vi "UMLEditor Main.vi"(1 "StartProject":string, 3 "StartTarget":string) -> ()   [LabVIEW 2012] (continued)
            n1211 = event-data() -> ()  [unwired: 2 out]
            n1212 = Unbundle By Name(w3369) -> ("ToolHelp"=w3371:bool)
            n1213 = local read "Help"() -> (w3370:bool)
            n1214 = And(x=w3371, y=w3370) -> (x .and. y?=w3368:bool)
            n1215 = case shown="True" w3368 {
              tunnel: w3373 -> [w3374 w3376]
              tunnel: [w3374 w3375] -> w3372
              tunnel: w3369 -> [_ _]
              frame False {
              }
              frame True {
                n1216 = call <resource>:"ContextHelp_HelpTexts.vi"("HelpText (enum or string)"=ContextHelp_HelpTexts."BClass" ("HelpText")) -> ("HelpOut"=w3378:T57)  [unwired: 18 out]
                n1217 = call <resource>:"ContextHelp_SendMessageToPopUp.vi"("PopUpMessage"=w3378, "error in (no error)"=w3376) -> ("error out"=w3375:errorcluster)  [unwired: 1 in, 16 out]
              }
            }
          }
          event Mouse Enter {
            n1218 = event-data() -> ()  [unwired: 2 out]
            n1219 = Unbundle By Name(w3379) -> ("ToolHelp"=w3382:bool)
            n1220 = local read "Help"() -> (w3381:bool)
            n1221 = And(x=w3382, y=w3381) -> (x .and. y?=w3380:bool)
            n1222 = case shown="True" w3380 {
              tunnel: w3384 -> [w3385 w3387]
              tunnel: [w3385 w3386] -> w3383
              tunnel: w3379 -> [_ _]
              frame False {
              }
              frame True {
                n1223 = call <resource>:"ContextHelp_HelpTexts.vi"("HelpText (enum or string)"=ContextHelp_HelpTexts."BInterface" ("HelpText")) -> ("HelpOut"=w3389:T57)  [unwired: 18 out]
                n1224 = call <resource>:"ContextHelp_SendMessageToPopUp.vi"("PopUpMessage"=w3389, "error in (no error)"=w3387) -> ("error out"=w3386:errorcluster)  [unwired: 1 in, 16 out]
              }
            }
          }
          event Mouse Enter {
            n1225 = event-data() -> ()  [unwired: 2 out]
            n1226 = Unbundle By Name(w3391) -> ("ToolHelp"=w3393:bool)
            n1227 = local read "Help"() -> (w3392:bool)
            n1228 = And(x=w3393, y=w3392) -> (x .and. y?=w3390:bool)
            n1229 = case shown="True" w3390 {
              tunnel: w3395 -> [w3396 w3398]
              tunnel: [w3396 w3397] -> w3394
              tunnel: w3391 -> [_ _]
              frame False {
              }
              frame True {
                n1230 = call <resource>:"ContextHelp_HelpTexts.vi"("HelpText (enum or string)"=ContextHelp_HelpTexts."BPackage" ("HelpText")) -> ("HelpOut"=w3400:T57)  [unwired: 18 out]
                n1231 = call <resource>:"ContextHelp_SendMessageToPopUp.vi"("PopUpMessage"=w3400, "error in (no error)"=w3398) -> ("error out"=w3397:errorcluster)  [unwired: 1 in, 16 out]
              }
            }
          }
          event Mouse Enter {
            n1232 = event-data() -> ()  [unwired: 2 out]
            n1233 = Unbundle By Name(w3401) -> ("ToolHelp"=w3404:bool)
            n1234 = local read "Help"() -> (w3403:bool)
            n1235 = And(x=w3404, y=w3403) -> (x .and. y?=w3402:bool)
            n1236 = case shown="True" w3402 {
              tunnel: w3406 -> [w3407 w3409]
              tunnel: [w3407 w3408] -> w3405
              tunnel: w3401 -> [_ _]
              frame False {
              }
              frame True {
                n1237 = call <resource>:"ContextHelp_HelpTexts.vi"("HelpText (enum or string)"=ContextHelp_HelpTexts."BDependency" ("HelpText")) -> ("HelpOut"=w3411:T57)  [unwired: 18 out]
                n1238 = call <resource>:"ContextHelp_SendMessageToPopUp.vi"("PopUpMessage"=w3411, "error in (no error)"=w3409) -> ("error out"=w3408:errorcluster)  [unwired: 1 in, 16 out]
              }
            }
          }
          event Mouse Enter {
            n1239 = event-data() -> ()  [unwired: 2 out]
            n1240 = Unbundle By Name(w3412) -> ("ToolHelp"=w3415:bool)
            n1241 = local read "Help"() -> (w3414:bool)
            n1242 = And(x=w3415, y=w3414) -> (x .and. y?=w3413:bool)
            n1243 = case shown="True" w3413 {
              tunnel: w3417 -> [w3418 w3420]
              tunnel: [w3418 w3419] -> w3416
              tunnel: w3412 -> [_ _]
              frame False {
              }
              frame True {
                n1244 = call <resource>:"ContextHelp_HelpTexts.vi"("HelpText (enum or string)"=ContextHelp_HelpTexts."BInheritance" ("HelpText")) -> ("HelpOut"=w3422:T57)  [unwired: 18 out]
                n1245 = call <resource>:"ContextHelp_SendMessageToPopUp.vi"("PopUpMessage"=w3422, "error in (no error)"=w3420) -> ("error out"=w3419:errorcluster)  [unwired: 1 in, 16 out]
              }
            }
          }
          event Mouse Enter {
            n1246 = event-data() -> ()  [unwired: 2 out]
            n1247 = Unbundle By Name(w3423) -> ("ToolHelp"=w3426:bool)
            n1248 = local read "Help"() -> (w3425:bool)
            n1249 = And(x=w3426, y=w3425) -> (x .and. y?=w3424:bool)
            n1250 = case shown="True" w3424 {
              tunnel: w3428 -> [w3429 w3431]
              tunnel: [w3429 w3430] -> w3427
              tunnel: w3423 -> [_ _]
              frame False {
              }
              frame True {
                n1251 = call <resource>:"ContextHelp_HelpTexts.vi"("HelpText (enum or string)"=ContextHelp_HelpTexts."BInterfaceImplementation" ("HelpText")) -> ("HelpOut"=w3433:T57)  [unwired: 18 out]
                n1252 = call <resource>:"ContextHelp_SendMessageToPopUp.vi"("PopUpMessage"=w3433, "error in (no error)"=w3431) -> ("error out"=w3430:errorcluster)  [unwired: 1 in, 16 out]
              }
            }
          }
          event Mouse Enter {
            n1253 = event-data() -> ()  [unwired: 2 out]
            n1254 = Unbundle By Name(w3434) -> ("ToolHelp"=w3437:bool)
            n1255 = local read "Help"() -> (w3436:bool)
            n1256 = And(x=w3437, y=w3436) -> (x .and. y?=w3435:bool)
            n1257 = case shown="True" w3435 {
              tunnel: w3439 -> [w3440 w3442]
              tunnel: [w3440 w3441] -> w3438
              tunnel: w3434 -> [_ _]
              frame False {
              }
              frame True {
                n1258 = call <resource>:"ContextHelp_HelpTexts.vi"("HelpText (enum or string)"=ContextHelp_HelpTexts."BAssociation" ("HelpText")) -> ("HelpOut"=w3444:T57)  [unwired: 18 out]
                n1259 = call <resource>:"ContextHelp_SendMessageToPopUp.vi"("PopUpMessage"=w3444, "error in (no error)"=w3442) -> ("error out"=w3441:errorcluster)  [unwired: 1 in, 16 out]
              }
            }
          }
          event Mouse Enter {
            n1260 = event-data() -> ()  [unwired: 2 out]
            n1261 = Unbundle By Name(w3446) -> ("ToolHelp"=w3448:bool)
            n1262 = local read "Help"() -> (w3447:bool)
            n1263 = And(x=w3448, y=w3447) -> (x .and. y?=w3445:bool)
            n1264 = case shown="True" w3445 {
              tunnel: w3450 -> [w3451 w3453]
              tunnel: [w3451 w3452] -> w3449
              tunnel: w3446 -> [_ _]
              frame False {
              }
              frame True {
                n1265 = call <resource>:"ContextHelp_HelpTexts.vi"("HelpText (enum or string)"=ContextHelp_HelpTexts."BAggregation" ("HelpText")) -> ("HelpOut"=w3455:T57)  [unwired: 18 out]
                n1266 = call <resource>:"ContextHelp_SendMessageToPopUp.vi"("PopUpMessage"=w3455, "error in (no error)"=w3453) -> ("error out"=w3452:errorcluster)  [unwired: 1 in, 16 out]
              }
            }
          }
          event Mouse Enter {
            n1267 = event-data() -> ()  [unwired: 2 out]
            n1268 = Unbundle By Name(w3456) -> ("ToolHelp"=w3459:bool)
            n1269 = local read "Help"() -> (w3458:bool)
            n1270 = And(x=w3459, y=w3458) -> (x .and. y?=w3457:bool)
            n1271 = case shown="False" w3457 {
              tunnel: w3461 -> [w3462 w3464]
              tunnel: [w3462 w3463] -> w3460
              tunnel: w3456 -> [_ _]
              frame False {
              }
              frame True {
                n1272 = call <resource>:"ContextHelp_HelpTexts.vi"("HelpText (enum or string)"=ContextHelp_HelpTexts."BCompAggregation" ("HelpText")) -> ("HelpOut"=w3466:T57)  [unwired: 18 out]
                n1273 = call <resource>:"ContextHelp_SendMessageToPopUp.vi"("PopUpMessage"=w3466, "error in (no error)"=w3464) -> ("error out"=w3463:errorcluster)  [unwired: 1 in, 16 out]
              }
            }
          }
          event Mouse Enter {
            # "Object"
            n1274 = event-data() -> ()  [unwired: 3 out]
            n1275 = Unbundle By Name(w3468) -> ("ToolHelp"=w3470:bool)
            n1276 = local read "Help"() -> (w3469:bool)
            n1277 = And(x=w3470, y=w3469) -> (x .and. y?=w3467:bool)
            n1278 = case shown="True" w3467 {
              tunnel: w3472 -> [w3473 w3475]
              tunnel: [w3473 w3474] -> w3471
              tunnel: w3468 -> [_ _]
              frame False {
              }
              frame True {
                n1279 = call <resource>:"ContextHelp_HelpTexts.vi"("HelpText (enum or string)"=ContextHelp_HelpTexts."BSystem" ("HelpText")) -> ("HelpOut"=w3477:T57)  [unwired: 18 out]
                n1280 = call <resource>:"ContextHelp_SendMessageToPopUp.vi"("PopUpMessage"=w3477, "error in (no error)"=w3475) -> ("error out"=w3474:errorcluster)  [unwired: 1 in, 16 out]
              }
            }
          }
          event Mouse Enter {
            # "Object"
            n1281 = event-data() -> ()  [unwired: 3 out]
            n1282 = Unbundle By Name(w3479) -> ("ToolHelp"=w3481:bool)
            n1283 = local read "Help"() -> (w3480:bool)
            n1284 = And(x=w3481, y=w3480) -> (x .and. y?=w3478:bool)
            n1285 = case shown="True" w3478 {
              tunnel: w3483 -> [w3484 w3486]
              tunnel: [w3484 w3485] -> w3482
              tunnel: w3479 -> [_ _]
              frame False {
              }
              frame True {
                n1286 = call <resource>:"ContextHelp_HelpTexts.vi"("HelpText (enum or string)"=ContextHelp_HelpTexts."BActor" ("HelpText")) -> ("HelpOut"=w3488:T57)  [unwired: 18 out]
                n1287 = call <resource>:"ContextHelp_SendMessageToPopUp.vi"("PopUpMessage"=w3488, "error in (no error)"=w3486) -> ("error out"=w3485:errorcluster)  [unwired: 1 in, 16 out]
              }
            }
          }
          event Mouse Enter {
            # "Object"
            n1288 = event-data() -> ()  [unwired: 3 out]
            n1289 = Unbundle By Name(w3490) -> ("ToolHelp"=w3492:bool)
            n1290 = local read "Help"() -> (w3491:bool)
            n1291 = And(x=w3492, y=w3491) -> (x .and. y?=w3489:bool)
            n1292 = case shown="True" w3489 {
              tunnel: w3494 -> [w3495 w3497]
              tunnel: [w3495 w3496] -> w3493
              tunnel: w3490 -> [_ _]
              frame False {
              }
              frame True {
                n1293 = call <resource>:"ContextHelp_HelpTexts.vi"("HelpText (enum or string)"=ContextHelp_HelpTexts."BUseCase" ("HelpText")) -> ("HelpOut"=w3499:T57)  [unwired: 18 out]
                n1294 = call <resource>:"ContextHelp_SendMessageToPopUp.vi"("PopUpMessage"=w3499, "error in (no error)"=w3497) -> ("error out"=w3496:errorcluster)  [unwired: 1 in, 16 out]
              }
            }
          }
          event Mouse Enter {
            # "Object"
            n1295 = event-data() -> ()  [unwired: 3 out]
            n1296 = Unbundle By Name(w3501) -> ("ToolHelp"=w3503:bool)
            n1297 = local read "Help"() -> (w3502:bool)
            n1298 = And(x=w3503, y=w3502) -> (x .and. y?=w3500:bool)
            n1299 = case shown="True" w3500 {
              tunnel: w3505 -> [w3506 w3508]
              tunnel: [w3506 w3507] -> w3504
              tunnel: w3501 -> [_ _]
              frame False {
              }
              frame True {
                n1300 = call <resource>:"ContextHelp_HelpTexts.vi"("HelpText (enum or string)"=ContextHelp_HelpTexts."BUseCaseDiagramAssociation" ("HelpText")) -> ("HelpOut"=w3510:T57)  [unwired: 18 out]
                n1301 = call <resource>:"ContextHelp_SendMessageToPopUp.vi"("PopUpMessage"=w3510, "error in (no error)"=w3508) -> ("error out"=w3507:errorcluster)  [unwired: 1 in, 16 out]
              }
            }
          }
          event Mouse Enter {
            # "Object"
            n1302 = event-data() -> ()  [unwired: 3 out]
            n1303 = Unbundle By Name(w3512) -> ("ToolHelp"=w3514:bool)
            n1304 = local read "Help"() -> (w3513:bool)
            n1305 = And(x=w3514, y=w3513) -> (x .and. y?=w3511:bool)
            n1306 = case shown="True" w3511 {
              tunnel: w3516 -> [w3517 w3519]
              tunnel: [w3517 w3518] -> w3515
              tunnel: w3512 -> [_ _]
              frame False {
              }
              frame True {
                n1307 = call <resource>:"ContextHelp_HelpTexts.vi"("HelpText (enum or string)"=ContextHelp_HelpTexts."BIncludes" ("HelpText")) -> ("HelpOut"=w3521:T57)  [unwired: 18 out]
                n1308 = call <resource>:"ContextHelp_SendMessageToPopUp.vi"("PopUpMessage"=w3521, "error in (no error)"=w3519) -> ("error out"=w3518:errorcluster)  [unwired: 1 in, 16 out]
              }
            }
          }
          event Mouse Enter {
            # "Object"
            n1309 = event-data() -> ()  [unwired: 3 out]
            n1310 = Unbundle By Name(w3523) -> ("ToolHelp"=w3525:bool)
            n1311 = local read "Help"() -> (w3524:bool)
            n1312 = And(x=w3525, y=w3524) -> (x .and. y?=w3522:bool)
            n1313 = case shown="True" w3522 {
              tunnel: w3527 -> [w3528 w3530]
              tunnel: [w3528 w3529] -> w3526
              tunnel: w3523 -> [_ _]
              frame False {
              }
              frame True {
                n1314 = call <resource>:"ContextHelp_HelpTexts.vi"("HelpText (enum or string)"=ContextHelp_HelpTexts."BExtends" ("HelpText")) -> ("HelpOut"=w3532:T57)  [unwired: 18 out]
                n1315 = call <resource>:"ContextHelp_SendMessageToPopUp.vi"("PopUpMessage"=w3532, "error in (no error)"=w3530) -> ("error out"=w3529:errorcluster)  [unwired: 1 in, 16 out]
              }
            }
          }
          event Mouse Enter {
            # "Object"
            n1316 = event-data() -> ()  [unwired: 3 out]
            n1317 = Unbundle By Name(w3534) -> ("ToolHelp"=w3536:bool)
            n1318 = local read "Help"() -> (w3535:bool)
            n1319 = And(x=w3536, y=w3535) -> (x .and. y?=w3533:bool)
            n1320 = case shown="True" w3533 {
              tunnel: w3538 -> [w3539 w3541]
              tunnel: [w3539 w3540] -> w3537
              tunnel: w3534 -> [_ _]
              frame False {
              }
              frame True {
                n1321 = call <resource>:"ContextHelp_HelpTexts.vi"("HelpText (enum or string)"=ContextHelp_HelpTexts."BGeneralization" ("HelpText")) -> ("HelpOut"=w3543:T57)  [unwired: 18 out]
                n1322 = call <resource>:"ContextHelp_SendMessageToPopUp.vi"("PopUpMessage"=w3543, "error in (no error)"=w3541) -> ("error out"=w3540:errorcluster)  [unwired: 1 in, 16 out]
              }
            }
          }
          event Mouse Enter {
            # "Object"
            n1323 = event-data() -> ()  [unwired: 3 out]
            n1324 = Unbundle By Name(w3545) -> ("ToolHelp"=w3547:bool)
            n1325 = local read "Help"() -> (w3546:bool)
            n1326 = And(x=w3547, y=w3546) -> (x .and. y?=w3544:bool)
            n1327 = case shown="True" w3544 {
              tunnel: w3549 -> [w3550 w3552]
              tunnel: [w3550 w3551] -> w3548
              tunnel: w3545 -> [_ _]
              frame False {
              }
              frame True {
                n1328 = call <resource>:"ContextHelp_HelpTexts.vi"("HelpText (enum or string)"=ContextHelp_HelpTexts."BObject" ("HelpText")) -> ("HelpOut"=w3554:T57)  [unwired: 18 out]
                n1329 = call <resource>:"ContextHelp_SendMessageToPopUp.vi"("PopUpMessage"=w3554, "error in (no error)"=w3552) -> ("error out"=w3551:errorcluster)  [unwired: 1 in, 16 out]
              }
            }
          }
          event Mouse Enter {
            # "Object"
            n1330 = event-data() -> ()  [unwired: 3 out]
            n1331 = Unbundle By Name(w3556) -> ("ToolHelp"=w3558:bool)
            n1332 = local read "Help"() -> (w3557:bool)
            n1333 = And(x=w3558, y=w3557) -> (x .and. y?=w3555:bool)
            n1334 = case shown="True" w3555 {
              tunnel: w3560 -> [w3561 w3563]
              tunnel: [w3561 w3562] -> w3559
              tunnel: w3556 -> [_ _]
              frame False {
              }
              frame True {
                n1335 = call <resource>:"ContextHelp_HelpTexts.vi"("HelpText (enum or string)"=ContextHelp_HelpTexts."BActionBar" ("HelpText")) -> ("HelpOut"=w3565:T57)  [unwired: 18 out]
                n1336 = call <resource>:"ContextHelp_SendMessageToPopUp.vi"("PopUpMessage"=w3565, "error in (no error)"=w3563) -> ("error out"=w3562:errorcluster)  [unwired: 1 in, 16 out]
              }
            }
          }
          event Mouse Enter {
            # "Object"
            n1337 = event-data() -> ()  [unwired: 3 out]
            n1338 = Unbundle By Name(w3567) -> ("ToolHelp"=w3569:bool)
            n1339 = local read "Help"() -> (w3568:bool)
            n1340 = And(x=w3569, y=w3568) -> (x .and. y?=w3566:bool)
            n1341 = case shown="True" w3566 {
              tunnel: w3571 -> [w3572 w3574]
              tunnel: [w3572 w3573] -> w3570
              tunnel: w3567 -> [_ _]
              frame False {
              }
              frame True {
                n1342 = call <resource>:"ContextHelp_HelpTexts.vi"("HelpText (enum or string)"=ContextHelp_HelpTexts."BCall" ("HelpText")) -> ("HelpOut"=w3576:T57)  [unwired: 18 out]
                n1343 = call <resource>:"ContextHelp_SendMessageToPopUp.vi"("PopUpMessage"=w3576, "error in (no error)"=w3574) -> ("error out"=w3573:errorcluster)  [unwired: 1 in, 16 out]
              }
            }
          }
          event Mouse Enter {
            n1344 = event-data() -> ()  [unwired: 2 out]
            n1345 = Unbundle By Name(w3577) -> ("ToolHelp"=w3580:bool)
            n1346 = local read "Help"() -> (w3579:bool)
            n1347 = And(x=w3580, y=w3579) -> (x .and. y?=w3578:bool)
            n1348 = case shown="True" w3578 {
              tunnel: w3582 -> [w3583 w3585]
              tunnel: [w3583 w3584] -> w3581
              tunnel: w3577 -> [_ _]
              frame False {
              }
              frame True {
                n1349 = call <resource>:"ContextHelp_HelpTexts.vi"("HelpText (enum or string)"=ContextHelp_HelpTexts."BNoteConnector" ("HelpText")) -> ("HelpOut"=w3587:T57)  [unwired: 18 out]
                n1350 = call <resource>:"ContextHelp_SendMessageToPopUp.vi"("PopUpMessage"=w3587, "error in (no error)"=w3585) -> ("error out"=w3584:errorcluster)  [unwired: 1 in, 16 out]
              }
            }
          }
          event Mouse Enter {
            n1351 = event-data() -> ()  [unwired: 4 out]
            n1352 = Unbundle By Name(w3588) -> ("ToolHelp"=w3593:bool)
            n1353 = local read "Help"() -> (w3592:bool)
            n1354 = And(x=w3593, y=w3592) -> (x .and. y?=w3591:bool)
            n1355 = case shown="True" w3591 {
              tunnel: w3589 -> [w3594 w3596]
              tunnel: [w3594 w3595] -> w3590
              tunnel: w3588 -> [_ _]
              frame False {
              }
              frame True {
                n1356 = call <resource>:"ContextHelp_HelpTexts.vi"("HelpText (enum or string)"=ContextHelp_HelpTexts."BNote" ("HelpText")) -> ("HelpOut"=w3598:T57)  [unwired: 18 out]
                n1357 = call <resource>:"ContextHelp_SendMessageToPopUp.vi"("PopUpMessage"=w3598, "error in (no error)"=w3596) -> ("error out"=w3595:errorcluster)  [unwired: 1 in, 16 out]
              }
            }
          }
          event Mouse Enter {
            n1358 = event-data() -> ()  [unwired: 4 out]
            n1359 = Unbundle By Name(w3599) -> ("ToolHelp"=w3604:bool)
            n1360 = local read "Help"() -> (w3603:bool)
            n1361 = And(x=w3604, y=w3603) -> (x .and. y?=w3602:bool)
            n1362 = case shown="True" w3602 {
              tunnel: w3600 -> [w3605 w3607]
              tunnel: [w3605 w3606] -> w3601
              tunnel: w3599 -> [_ _]
              frame False {
              }
              frame True {
                n1363 = call <resource>:"ContextHelp_HelpTexts.vi"("HelpText (enum or string)"=ContextHelp_HelpTexts."BState" ("HelpText")) -> ("HelpOut"=w3609:T57)  [unwired: 18 out]
                n1364 = call <resource>:"ContextHelp_SendMessageToPopUp.vi"("PopUpMessage"=w3609, "error in (no error)"=w3607) -> ("error out"=w3606:errorcluster)  [unwired: 1 in, 16 out]
              }
            }
          }
          event Mouse Enter {
            n1365 = event-data() -> ()  [unwired: 4 out]
            n1366 = Unbundle By Name(w3610) -> ("ToolHelp"=w3615:bool)
            n1367 = local read "Help"() -> (w3614:bool)
            n1368 = And(x=w3615, y=w3614) -> (x .and. y?=w3613:bool)
            n1369 = case shown="True" w3613 {
              tunnel: w3611 -> [w3616 w3618]
              tunnel: [w3616 w3617] -> w3612
              tunnel: w3610 -> [_ _]
              frame False {
              }
              frame True {
                n1370 = call <resource>:"ContextHelp_HelpTexts.vi"("HelpText (enum or string)"=ContextHelp_HelpTexts."BInitialState" ("HelpText")) -> ("HelpOut"=w3620:T57)  [unwired: 18 out]
                n1371 = call <resource>:"ContextHelp_SendMessageToPopUp.vi"("PopUpMessage"=w3620, "error in (no error)"=w3618) -> ("error out"=w3617:errorcluster)  [unwired: 1 in, 16 out]
              }
            }
          }
          event Mouse Enter {
            n1372 = event-data() -> ()  [unwired: 4 out]
            n1373 = Unbundle By Name(w3621) -> ("ToolHelp"=w3626:bool)
            n1374 = local read "Help"() -> (w3625:bool)
            n1375 = And(x=w3626, y=w3625) -> (x .and. y?=w3624:bool)
            n1376 = case shown="True" w3624 {
              tunnel: w3622 -> [w3627 w3629]
              tunnel: [w3627 w3628] -> w3623
              tunnel: w3621 -> [_ _]
              frame False {
              }
              frame True {
                n1377 = call <resource>:"ContextHelp_HelpTexts.vi"("HelpText (enum or string)"=ContextHelp_HelpTexts."BFinalState" ("HelpText")) -> ("HelpOut"=w3631:T57)  [unwired: 18 out]
                n1378 = call <resource>:"ContextHelp_SendMessageToPopUp.vi"("PopUpMessage"=w3631, "error in (no error)"=w3629) -> ("error out"=w3628:errorcluster)  [unwired: 1 in, 16 out]
              }
            }
          }
          event Mouse Enter {
            n1379 = event-data() -> ()  [unwired: 4 out]
            n1380 = Unbundle By Name(w3632) -> ("ToolHelp"=w3637:bool)
            n1381 = local read "Help"() -> (w3636:bool)
            n1382 = And(x=w3637, y=w3636) -> (x .and. y?=w3635:bool)
            n1383 = case shown="True" w3635 {
              tunnel: w3633 -> [w3638 w3640]
              tunnel: [w3638 w3639] -> w3634
              tunnel: w3632 -> [_ _]
              frame False {
              }
              frame True {
                n1384 = call <resource>:"ContextHelp_HelpTexts.vi"("HelpText (enum or string)"=ContextHelp_HelpTexts."BStateTransition" ("HelpText")) -> ("HelpOut"=w3642:T57)  [unwired: 18 out]
                n1385 = call <resource>:"ContextHelp_SendMessageToPopUp.vi"("PopUpMessage"=w3642, "error in (no error)"=w3640) -> ("error out"=w3639:errorcluster)  [unwired: 1 in, 16 out]
              }
            }
          }
          event "RevHistory": Mouse Down {
            n1386 = event-data() -> ("Mods.Double Click"=w3643:bool)  [unwired: 1 out]
            n1387 = case shown="True" w3643 {
              tunnel: w3646 -> [w3647 w3650]
              tunnel: [w3647 w3649] -> w3645
              tunnel: w3644 -> [_ w3648]
              frame False {
              }
              frame True {
                n1388 = call <resource>:"UMLEditor RevisionHistory.vi"("localVariables"=w3648, "error in (no error)"=w3650) -> ("error out"=w3649:errorcluster)  [unwired: 17 out]
              }
            }
          }
          event "Project": Value Change {
            n1389 = event-data() -> ()  [unwired: 2 out]
            n1390 = property on="Project" class="Ring (strict)"() -> ("Strings []"=w3662:string[])  [unwired: 2 in, 2 out]
            n1391 = Index Array(array=w3662, index="Project") -> (element=w3655:string)
            n1392 = call <resource>:"UMLEditor_TargetDialog.vi"("error in (no error)"=w3656, "GetProjectRefByName"=w3655) -> ("error out"=w3653:errorcluster, "ProjectFolder"=w3654:path, "TargetIndex"=w3652:u16, "Targets"=w3651:string[])  [unwired: 5 in, 1 out]
            n1393 = call <resource>:"GetRelativePathOption.vi"() -> ("UseProjectFolderAsBasePath"=w3660:bool)  [unwired: 1 in, 18 out]
            n1394 = property on="Target" class="Ring (strict)"("Strings []"=w3651, "Value"=w3652) -> ()  [unwired: 2 in, 2 out]
            n1395 = case shown="True" w3660 {
              tunnel: w3654 -> [_ w3682]
              tunnel: File_StoredPathesActions."Set Path" ("Method (Get Path)") -> [_ w3681]
              frame False {
              }
              frame True {
                n1396 = call <resource>:"File_ApplicationPaths.vi"("PathName"=UMLEditor_StoredPathes."ClassBasePath" ("UMLPathes"), "Path In"=w3682, "Method (Get Path)"=w3681) -> ()  [unwired: 1 in, 16 out]
              }
            }
            n1397 = Unbundle By Name(w3653) -> ("code"=w3658:i32)
            n1398 = case shown="1055" w3658 {
              tunnel: w3653 -> [w3664 _]
              tunnel: [w3664 w3673] -> w3657
              tunnel: w3656 -> [_ w3673]
              frame 0, Default {
              }
              frame 1055 {
                n1399 = call <resource>:"GDSProject_GetProjects.vi"("OpenProjectRef(True)"=FALSE) -> ("Projects"=w3674:string[])  [unwired: 2 in, 16 out]
                n1400 = Index Array(array=w3674) -> (element=w3672:string)  [unwired: 1 in]
                n1401 = stacked-sequence {
                  tunnel: [w3679] -> w3671
                  tunnel: w3672 -> [w3679]
                  frame #0 {
                    n1402 = One Button Dialog(message="The selected project has been closed.\nSelect another one.") -> ()  [unwired: 2 out]
                  }
                }
                n1403 = call <resource>:"UMLEditor_TargetDialog.vi"("GetProjectRefByName"=w3671) -> ("ProjectFolder"=w3665:path, "TargetIndex"=w3670:u16, "Targets"=w3669:string[])  [unwired: 6 in, 2 out]
                n1404 = call <resource>:"GetRelativePathOption.vi"() -> ("UseProjectFolderAsBasePath"=w3667:bool)  [unwired: 1 in, 18 out]
                n1405 = case shown="True" w3667 {
                  tunnel: w3665 -> [_ w3677]
                  tunnel: File_StoredPathesActions."Set Path" ("Method (Get Path)") -> [_ w3676]
                  frame False {
                  }
                  frame True {
                    n1406 = call <resource>:"File_ApplicationPaths.vi"("PathName"=UMLEditor_StoredPathes."ClassBasePath" ("UMLPathes"), "Path In"=w3677, "Method (Get Path)"=w3676) -> ()  [unwired: 1 in, 16 out]
                  }
                }
                n1407 = property on="Project" class="Ring (strict)"("Strings []"=w3674, "Value"=0) -> ()  [unwired: 2 in, 2 out]
                n1408 = property on="Target" class="Ring (strict)"("Strings []"=w3669, "Value"=w3670) -> ()  [unwired: 2 in, 2 out]
              }
            }
          }
          event "Project": Mouse Down? {
            n1409 = event-data() -> ()  [unwired: 2 out]
            n1410 = property on="Project" class="Ring (strict)"() -> ("Strings []"=w3685:string[])  [unwired: 2 in, 2 out]
            n1411 = call <resource>:"UMLEditor getDiagramInfo.vi"("localVariables"=w3694, "error in (no error)"=w3692) -> ("graph"=w3691:refnum<class "Graph.lvclass">, "error out"=w3690:errorcluster)  [unwired: 16 out]
            n1412 = Index Array(array=w3685) -> (element=w3687:string)  [unwired: 1 in]
            n1413 = Empty String/Path?(string/path=w3687) -> (empty?=w3686:bool)
            n1414 = call-dynamic "getNodes.vi"("reference"=w3691, "error in (no error)"=w3690) -> ("nodes"=w3689:refnum<class "AbstractNode.lvclass">[])  [unwired: 15 in, 2 out]
            n1415 = Empty Array?(array=w3689) -> (empty?=w3688:bool)
            n1416 = Or(x=w3688, y=w3686) -> ()  [unwired: 1 out]
            n1417 = case shown="True" TRUE {
              tunnel: w3692 -> [w3697 w3706]
              tunnel: [w3697 w3705] -> w3695
              tunnel: [TRUE ("Discard?") w3704] -> w3693
              tunnel: w3685 -> [_ w3701]
              frame False {
                n1418 = One Button Dialog(message="You are only allowed to change project if the current diagram is empty.") -> ()  [unwired: 2 out]
              }
              frame True {
                n1419 = call <resource>:"GDSProject_GetProjects.vi"("error in (no error)"=w3706, "OpenProjectRef(True)"=FALSE) -> ("Projects"=w3700:string[], "error out"=w3705:errorcluster)  [unwired: 1 in, 15 out]
                n1420 = Index Array(array=w3700) -> (element=w3703:string)  [unwired: 1 in]
                n1421 = Empty String/Path?(string/path=w3703) -> (empty?=w3702:bool)
                n1422 = case shown="True" w3702 {
                  tunnel: [FALSE ("Discard?") TRUE ("Discard?")] -> w3704
                  tunnel: w3700 -> [w3709 _]
                  tunnel: w3701 -> [w3708 _]
                  frame False {
                    n1423 = for {
                      tunnel: w3709 -> [w3711] mode=indexing
                      shift-right: [w3714] -> w3707
                      shift-left: w3708 -> [w3713]
                      n1424 = Search 1D Array(1D array=w3713, element=w3711) -> (index of element=w3712:i32)  [unwired: 1 out]
                      n1425 = case shown="0, Default" w3712 {
                        tunnel: [w3715 w3718] -> w3714
                        tunnel: w3713 -> [w3715 w3717]
                        tunnel: w3711 -> [_ w3716]
                        frame 0, Default {
                        }
                        frame -1 {
                          n1426 = Build Array (concatenate)(w3717, w3716) -> (w3718:string[])
                        }
                      }
                    }
                    n1427 = property on="Project" class="Ring (strict)"("Strings []"=w3707) -> ()  [unwired: 2 in, 2 out]
                  }
                  frame True {
                    n1428 = call "File Dialog"("prompt"="Select a project to open", "button label"="Open", "pattern (all files)"="*.lvproj", "pattern label"="LabVIEW projects") -> ("selected path"=w3719:path, "cancelled"=w3720:bool)  [unwired: 3 in, 7 out]
                    n1429 = case shown="False" w3720 {
                      tunnel: w3719 -> [w3741 _]
                      frame False {
                        n1430 = call <vilib>:"Set Busy.vi"() -> ("error out"=w3735:errorcluster)  [unwired: 4 in, 7 out]
                        n1431 = invoke class="App" method="Project.Open"(error in=w3735, "Path"=w3741) -> ("Project:Open"=w3740:refnum<vi>)  [unwired: 2 in, 3 out]
                        n1432 = invoke class="Project" method="Open Window"(reference=w3740) -> (reference out=w3738:refnum<vi>, error out=w3739:errorcluster)  [unwired: 2 in, 1 out]
                        n1433 = call <resource>:"GetRelativePathOption.vi"() -> ("UseProjectFolderAsBasePath"=w3728:bool)  [unwired: 1 in, 18 out]
                        n1434 = Close Reference(reference=w3738, error in (no error)=w3739) -> (error out=w3737:errorcluster)
                        n1435 = call <resource>:"GDSProject_GetProjects.vi"("error in (no error)"=w3737, "OpenProjectRef(True)"=FALSE) -> ("Projects"=w3736:string[])  [unwired: 1 in, 16 out]
                        n1436 = Index Array(array=w3736) -> (element=w3733:string)  [unwired: 1 in]
                        n1437 = call <resource>:"UMLEditor_TargetDialog.vi"("GetProjectRefByName"=w3733) -> ("error out"=w3732:errorcluster, "ProjectFolder"=w3726:path, "TargetIndex"=w3730:u16, "Targets"=w3731:string[])  [unwired: 6 in, 1 out]
                        n1438 = case shown="True" w3728 {
                          tunnel: w3726 -> [_ w3743]
                          tunnel: File_StoredPathesActions."Set Path" ("Method (Get Path)") -> [_ w3742]
                          frame False {
                          }
                          frame True {
                            n1439 = call <resource>:"File_ApplicationPaths.vi"("PathName"=UMLEditor_StoredPathes."ClassBasePath" ("UMLPathes"), "Path In"=w3743, "Method (Get Path)"=w3742) -> ()  [unwired: 1 in, 16 out]
                          }
                        }
                        n1440 = property on="Target" class="Ring (strict)"("Strings []"=w3731, "Value"=w3730) -> ()  [unwired: 2 in, 2 out]
                        n1441 = Build Array(w3733) -> (w3734:string[])
                        n1442 = property on="Project" class="Ring (strict)"("Strings []"=w3734) -> ()  [unwired: 2 in, 2 out]
                        n1443 = call <vilib>:"Unset Busy.vi"("error in (no error)"=w3732) -> ()  [unwired: 1 in, 10 out]
                      }
                      frame True {
                      }
                    }
                  }
                }
              }
            }
            n1444 = event-data("Discard?"=w3693) -> ()  [unwired: 1 in, 1 out]
          }
          event "ClassAggregationDialog": Value Change {
            n1445 = event-data() -> ()  [unwired: 7 out]
            n1446 = Unbundle By Name("ClassAggregationDialog") -> ("AddAttribute"=w3745:bool)  [unwired: 1 out]
            n1447 = property on="ClassAggregationDialog" class="Clust (strict)"("Visible"=FALSE) -> ()  [unwired: 2 in, 2 out]
            n1448 = call <resource>:"UMLEditor_AggregationClusterDialogControl.vi"("error in (no error)"=w3750, "Action(SelectSelect)"=T22."GetStatus") -> ("StartEndNodes"=w3747:T59, "AddAggregate?"=w3748:bool, "error out"=w3749:errorcluster)  [unwired: 7 in, 8 out]
            n1449 = case shown="True" w3745 {
              tunnel: w3754 -> [w3759 w3769]
              tunnel: w3749 -> [w3760 w3770]
              tunnel: [w3760 w3763] -> w3755
              tunnel: [w3759 w3768] -> w3753
              tunnel: w3752 -> [_ w3765]
              tunnel: w3748 -> [_ w3762]
              tunnel: w3747 -> [_ w3761]
              frame False {
              }
              frame True {
                n1450 = case shown="False" w3762 {
                  tunnel: w3770 -> [w3775 w3781]
                  tunnel: w3769 -> [w3774 w3782]
                  tunnel: [w3773 w3778] -> w3767
                  tunnel: [w3772 w3779] -> w3766
                  tunnel: [w3771 w3780] -> w3764
                  tunnel: w3761 -> [_ w3777]
                  frame True {
                    n1451 = Unbundle By Name(w3774) -> ("selectedEdge"=w3776:refnum<class "AbstractEdge.lvclass">)
                    n1452 = call <resource>:"UMLEditor CreateAggregationAttributes.vi"("ClassAggregation"=w3776, "error in (no error)"=w3775) -> ("NodeModified"=w3771:refnum<class "AbstractNode.lvclass">, "Modified?"=w3773:bool, "error out"=w3772:errorcluster)  [unwired: 15 out]
                  }
                  frame False {
                    n1453 = Unbundle By Name(w3782) -> ()  [unwired: 1 out]
                    n1454 = call <resource>:"UMLEditor RemoveAggregationAttributes.vi"("StartEndNodes"=w3777, "error in (no error)"=w3781) -> ("NodeModified"=w3780:refnum<class "AbstractNode.lvclass">, "Modified?"=w3778:bool, "error out"=w3779:errorcluster)  [unwired: 15 out]
                  }
                }
                n1455 = case shown="True" w3767 {
                  tunnel: w3769 -> [w3784 w3794]
                  tunnel: [w3784 w3793] -> w3768
                  tunnel: w3766 -> [w3783 w3791]
                  tunnel: w3765 -> [_ w3790]
                  tunnel: w3764 -> [_ w3789]
                  tunnel: [w3783 w3786] -> w3763
                  frame False {
                  }
                  frame True {
                    n1456 = Build Array(w3789) -> (w3788:refnum<class "AbstractNode.lvclass">[])
                    n1457 = call-dynamic "layout.vi"("reference"=w3790, "LayoutNodes(Empty=All)"=w3788, "error in (no error)"=w3791) -> ("error out"=w3787:errorcluster)  [unwired: 15 in, 1 out]
                    n1458 = Bundle By Name(cluster=w3794, "modified"=TRUE, "state"=UMLEditor_statesType."Repaint") -> (w3785:T7)
                    n1459 = call <resource>:"UMLEditor setDiagramInfo.vi"("error in (no error)"=w3787, "localVariablesIn"=w3785, "action"=enum16{"Name/Dir", "Unsaved", "Saved"}."Unsaved") -> ("localVariablesOut"=w3793:T7, "error out"=w3786:errorcluster)  [unwired: 2 in, 13 out]
                  }
                }
              }
            }
            n1460 = stacked-sequence {
              tunnel: [T5 {"AddAttribute"=FALSE, "Don'tAddAttribute"=FALSE, "Close"=FALSE, "Text"=""} ("ClassAggregationDialog")] -> w3746
              tunnel: w3745 -> [_]
              frame #0 {
              }
            }
            n1461 = local write "ClassAggregationDialog"(w3746) -> ()
          }
          event "Target": Value Change {
            n1462 = event-data() -> ()  [unwired: 7 out]
            n1463 = property on="Target" class="Ring (strict)"() -> ("Strings []"=w3805:string[], "Value"=w3804:u16)  [unwired: 2 in, 2 out]
            n1464 = property on="Project" class="Ring (strict)"() -> ("Strings []"=w3800:string[], "Value"=w3799:u16)  [unwired: 2 in, 2 out]
            n1465 = Index Array(array=w3805, index=w3804) -> (element=w3803:string)
            n1466 = Index Array(array=w3800, index=w3799) -> (element=w3798:string)
            n1467 = call <resource>:"UMLEditor_TargetDialog.vi"("error in (no error)"=w3802, "Target"=w3803, "GetProjectRefByName"=w3798) -> ("error out"=w3801:errorcluster)  [unwired: 4 in, 4 out]
          }
        }
        n1468 = Unbundle By Name(w278) -> ("Sync"=w270:bool, "state"=w268:T8)
        n1469 = Select(t=UMLEditor_statesType."AutoSync" ("state"), s=w270, f=w268) -> (s? t:f=w269:T8)
      }
      frame "AutoSync" {
        (unwired) UMLEditor_statesType."Idle" ("state")
        # "Have we been idle for a while?\nIf so, do a sync"
        n1470 = Unbundle By Name(w3809) -> ("LastSync"=w3816:timestamp, "SyncTime"=w3815:u32, "ForceSyncNow"=w3817:bool)
        n1471 = Get Date/Time In Seconds() -> (seconds since 1Jan1904=w3807:timestamp)
        n1472 = Subtract(x=w3807, y=w3816) -> (x-y=w3814:dbl)
        n1473 = Subtract(x=w3815, y=w3814) -> (x-y=w3813:dbl)
        n1474 = To Long Integer(number=w3813) -> (32bit integer=w3810:i32)
        n1475 = Max & Min(x=0, y=w3810) -> (max(x,y)=w3806:i32)  [unwired: 1 out]
        n1476 = Equal To 0?(x=w3806) -> (x = 0?=w3811:bool)
        n1477 = Or(x=w3811, y=w3817) -> (x .or. y?=w3818:bool)
        n1478 = case shown="False" w3818 {
          tunnel: w3824 -> [_ _]
          tunnel: w3809 -> [_ w3855]
          tunnel: [_ w3839] -> w3823
          tunnel: w3817 -> [_ w3840]
          tunnel: w3806 -> [w3827 _]
          tunnel: w3809 -> [w3826 w3838]
          tunnel: [w3826 w3837] -> w3808
          tunnel: w3807 -> [_ w3836]
          frame False {
            n1479 = feedback-in #2(w3827) -> ()
            n1480 = feedback #2() -> (w3829:i32)  [unwired: 1 in]
            n1481 = Not Equal?(x=w3829, y=w3827) -> (x != y?=w3828:bool)
            n1482 = case shown="True" w3828 {
              tunnel: w3827 -> [_ w3830]
              frame False {
              }
              frame True {
                n1483 = case shown="1" w3830 {
                  selector: w3830 -> [_ w3833]
                  tunnel: ["Auto sync in 1 second" ("format string") w3834] -> w3831
                  frame 1 {
                  }
                  frame Default {
                    n1484 = Format Into String(format string="Auto sync in %d seconds", w3833) -> (resulting string=w3834:string)  [unwired: 2 in, 1 out]
                  }
                }
                n1485 = local write "StatusBar"(w3831) -> ()
              }
            }
          }
          frame True {
            w3845 = timestamp(0 s since 1904-01-01)
            n1486 = call <resource>:"UMLEditor getDiagramInfo.vi"("localVariables"=w3855) -> ("graph"=w3841:refnum<class "Graph.lvclass">)  [unwired: 1 in, 17 out]
            n1487 = call-dynamic "getNodes.vi"("reference"=w3841) -> ("nodes"=w3856:refnum<class "AbstractNode.lvclass">[])  [unwired: 16 in, 2 out]
            n1488 = Bundle By Name(cluster=w3838, "LastSync"=w3836) -> (w3837:T7)
            n1489 = for {
              tunnel: w3856 -> [w3889] mode=indexing
              shift-right: [w3884] -> w3853
              shift-left: path[] [] -> [w3885]
              w3888 = refnum<class "ClassNode.lvclass"> refnum  # ClassNode.lvclass
              n1490 = To More Specific Class(target class=w3888, reference=w3889) -> (specific class reference=w3887:refnum<class "ClassNode.lvclass">, error out=w3886:errorcluster)  [unwired: 1 in]
              n1491 = case shown="No Error" w3886 {
                selector: w3886 -> [w3894 _]
                tunnel: w3887 -> [w3895 _]
                tunnel: w3885 -> [w3892 w3900]
                tunnel: [w3891 w3900] -> w3884
                frame No Error {
                  n1492 = call-dynamic "getClassInfo.vi"("reference"=w3895, "error in (no error)"=w3894) -> ("ClassPath"=w3890:path)  [unwired: 8 in, 9 out]
                  n1493 = Empty String/Path?(string/path=w3890) -> (empty?=w3893:bool)
                  n1494 = case shown="True" w3893 {
                    tunnel: w3892 -> [w3898 w3899]
                    tunnel: [w3897 w3899] -> w3891
                    tunnel: w3890 -> [w3896 _]
                    frame False {
                      n1495 = Build Array (concatenate)(w3898, w3896) -> (w3897:path[])
                    }
                    frame True {
                    }
                  }
                }
                frame Error {
                }
              }
            }
            n1496 = for {
              tunnel: w3853 -> [w3872] mode=indexing
              tunnel: path[] [path "Protected/ObjectAttributes.ctl", path "ObjectAttributes.ctl"] -> [w3871]
              shift-right: [w3865] -> w3843
              shift-left: w3845 -> [w3866]
              shift-right: [w3864] -> w3847
              shift-left: w3845 -> [w3862]
              shift-right: [w3859] -> w3846
              shift-left: w3845 -> [w3861]
              n1497 = Strip Path(path=w3872) -> (stripped path=w3870:path)  [unwired: 1 out]
              n1498 = List Folder(path=w3870, pattern="*.vi") -> (path out=w3867:path, filenames=w3869:string[])  [unwired: 2 in, 2 out]
              n1499 = File/Directory Info(path=w3872) -> (last mod=w3860:timestamp)  [unwired: 1 in, 6 out]
              n1500 = for {
                tunnel: w3870 -> [w3883]
                tunnel: w3871 -> [w3882] mode=indexing
                tunnel: [w3879] -> w3863
                stop <- w3880 continue-if-true
                n1501 = Build Path(base path=w3883, name or relative path=w3882) -> (appended path=w3881:path)
                n1502 = File/Directory Info(path=w3881) -> (last mod=w3879:timestamp, error out=w3880:errorcluster)  [unwired: 1 in, 5 out]
              }
              n1503 = for {
                tunnel: w3869 -> [w3877] mode=indexing
                tunnel: w3867 -> [w3878]
                shift-right: [w3873] -> w3865
                shift-left: w3866 -> [w3874]
                n1504 = Build Path(base path=w3878, name or relative path=w3877) -> (appended path=w3876:path)
                n1505 = File/Directory Info(path=w3876) -> (last mod=w3875:timestamp)  [unwired: 1 in, 6 out]
                n1506 = Max & Min(x=w3874, y=w3875) -> (max(x,y)=w3873:timestamp)  [unwired: 1 out]
              }
              n1507 = Max & Min(x=w3862, y=w3863) -> (max(x,y)=w3864:timestamp)  [unwired: 1 out]
              n1508 = Max & Min(x=w3861, y=w3860) -> (max(x,y)=w3859:timestamp)  [unwired: 1 out]
            }
            n1509 = feedback-in #3(w3843) -> ()
            n1510 = feedback #3() -> (w3844:timestamp)  [unwired: 1 in]
            n1511 = feedback-in #4(w3847) -> ()
            n1512 = feedback #4() -> (w3851:timestamp)  [unwired: 1 in]
            n1513 = feedback-in #5(w3846) -> ()
            n1514 = feedback #5() -> (w3852:timestamp)  [unwired: 1 in]
            n1515 = Not Equal?(x=w3843, y=w3844) -> (x != y?=w3842:bool)
            n1516 = Not Equal?(x=w3847, y=w3851) -> (x != y?=w3850:bool)
            n1517 = Not Equal?(x=w3846, y=w3852) -> (x != y?=w3849:bool)
            n1518 = Compound Arithmetic op=OR(w3840, w3842, w3850, w3849) -> (w3839:bool)
            n1519 = case shown="False" w3839 {
              frame False {
                n1520 = Wait (ms)(milliseconds to wait=u32 1000) -> ()  [unwired: 1 out]
                n1521 = local write "StatusBar"("No sync needed, no change was found" ("StatusBar")) -> ()
              }
              frame True {
              }
            }
          }
        }
        n1522 = Bundle By Name(cluster=w3808, "ForceSyncNow"=FALSE ("Sync")) -> (w3820:T7)
        n1523 = Unbundle By Name(w3820) -> ("state"=w3821:T8)
        n1524 = Select(t=UMLEditor_statesType."SyncAll" ("state"), s=w3823, f=w3821) -> (s? t:f=w3825:T8)
      }
      frame "AddNodeFromProjectTree", "AddNodeFromProjectTree+SyncAll" {
        n1525 = call <resource>:"CommonVIs_UmlOpenVIRef.vi"("error in"=w3930) -> ("error out"=w3929:errorcluster, "ProjectNameOut"=w3928:string)  [unwired: 3 in, 6 out]
        n1526 = property on="Picture" class="Pict"() -> ("Mouse"=w3919:T42)  [unwired: 2 in, 2 out]
        n1527 = Unbundle By Name(w3919) -> ("Mouse Position"=w3916:cluster{"X":i32, "Y":i32})
        n1528 = Unbundle By Name(w3915) -> ("zoom"=w3920:dbl, "offset"=w3917:T12)
        n1529 = call <resource>:"GDSProject_GetProjects.vi"("GetProjectRefByName"=w3928, "error in (no error)"=w3929) -> ("Project Refnum"=w3926:refnum<vi>, "error out"=w3927:errorcluster)  [unwired: 1 in, 15 out]
        n1530 = property class="Project"(reference=w3926, error in=w3927) -> (reference out=w3912:refnum<vi>, error out=w3922:errorcluster, "Selected Items in Tree"=w3925:refnum<vi>[], "Window State"=w3901:T60)
        n1531 = Add(x=w3917, y=w3916) -> (x+y=w3918:T12)
        n1532 = Empty Array?(array=w3925) -> (empty?=w3913:bool)
        n1533 = Close Reference(reference=w3912) -> (error out=w3911:errorcluster)  [unwired: 1 in]
        n1534 = Divide(x=w3918, y=w3920) -> (x/y=w3909:T12)
        n1535 = Max & Min(x=w3909, y=T12 {"x"=0.0, "y"=0.0}) -> (max(x,y)=w3907:T12)  [unwired: 1 out]
        n1536 = Unbundle(w3907) -> ("x"=w3906:dbl, "y"=w3905:dbl)
        n1537 = Max & Min(x=w3906, y=w3905) -> (max(x,y)=w3904:dbl)  [unwired: 1 out]
        n1538 = Less?(x=w3904, y=10.0) -> (x < y?=w3902:bool)
        n1539 = Or(x=w3902, y=w3913) -> (x .or. y?=w3914:bool)
        n1540 = case shown="False" w3914 {
          tunnel: w3925 -> [w3946 _]
          tunnel: w3915 -> [w3975 w4100]
          tunnel: [w3974 w4100] -> w3924
          tunnel: [w3971 w4097] -> w3923
          tunnel: w3915 -> [w3933 _]
          tunnel: w3922 -> [w3973 w4098]
          tunnel: [w3972 UMLEditor_statesType."Idle" ("state")] -> w3921
          tunnel: w3907 -> [w3965 _]
          tunnel: w3911 -> [_ _]
          tunnel: w3910 -> [w3942 _]
          tunnel: w3901 -> [_ _]
          frame False {
            # "Node Tool"
            n1541 = Index Array(array=w3946) -> (element=w3945:refnum<vi>)  [unwired: 1 in]
            n1542 = call <resource>:"UMLEditor getDiagramInfo.vi"("localVariables"=w3933, "error in (no error)"=w3973) -> ("graph"=w3941:refnum<class "Graph.lvclass">, "diagramType"=w3934:T11, "error out"=w3939:errorcluster)  [unwired: 15 out]
            n1543 = property class="ProjectItem" props=["Name", "Item ID", "Path", "Reference", "Library Item Type String"](reference=w3945) -> ("Name"=w3969:string, "Item ID"=w3966:string, "Path"=w3967:path, "Reference"=w3964:refnum<vi>)  [unwired: 1 in, 3 out]
            n1544 = Equal?(x=diagramType."Class" ("diagramType"), y=w3934) -> (x = y?=w3951:bool)
            n1545 = property class="VI"(reference=w3964) -> (reference out=w3953:refnum<vi>, error out=w3963:errorcluster, "Library"=w3962:refnum<vi>)  [unwired: 1 in]
            n1546 = call <resource>:"UMLEditor_GetAllClassNodeNames.vi"("error in"=w3939, "graph"=w3941) -> ("error out"=w3938:errorcluster, "ClassNodeNames(WithoutStereotype)"=w3937:string[])  [unwired: 8 out]
            n1547 = call <vilib>:"Get File Extension.vi"("file"=w3967) -> ("lowercase file extension"=w3948:string)  [unwired: 1 in, 9 out]
            n1548 = Empty String/Path?(string/path=w3948) -> (empty?=w3947:bool)
            n1549 = Not(x=w3947) -> (.not. x?=w3949:bool)
            n1550 = property class="Library"(reference=w3962, error in=w3963) -> (reference out=w3955:refnum<vi>, error out=w3956:errorcluster, "Name"=w3961:string)
            n1551 = Close Reference(reference=w3955, error in (no error)=w3956) -> (error out=w3954:errorcluster)
            n1552 = Close Reference(reference=w3953, error in (no error)=w3954) -> (error out=w3943:errorcluster)
            n1553 = Match Pattern(string=w3969, regular expression="\\.[~\\.]*$") -> (before substring=w3968:string)  [unwired: 4 out]
            n1554 = Match Pattern(string=w3961, regular expression="\\.[~\\.]*$") -> (before substring=w3958:string, offset past match=w3959:i32)  [unwired: 3 out]
            n1555 = case shown="0, Default" w3959 {
              tunnel: w3958 -> [w4085 _]
              tunnel: [w4084 _] -> w3957
              tunnel: w3943 -> [_ _]
              frame 0, Default {
                n1556 = Format Into String(format string="%s : ", w4085) -> (resulting string=w4084:string)  [unwired: 2 in, 1 out]
              }
              frame -1 {
              }
            }
            n1557 = case shown="\"vi\", \"vit\"" w3948 {
              tunnel: w3968 -> [w4087 w4091 w4093]
              tunnel: [w4088 w4092 w4093] -> w3940
              tunnel: w3966 -> [_ _ _]
              tunnel: w3957 -> [_ w4089 _]
              frame "vi", "vit" {
                n1558 = Concatenate Strings("<<VI>>\n" ("string"), w4087) -> (w4088:string)
              }
              frame "ctl", "ctt" {
                n1559 = Concatenate Strings("<<TYPE>>\n" ("string"), w4089, w4091) -> (w4092:string)
              }
              frame Default {
              }
            }
            n1560 = call <resource>:"CommonVIs SterotypeStringParser.vi"("SterotypeStringIn"=w3940) -> ("Name"=w3936:string)  [unwired: 18 out]
            n1561 = Search 1D Array(1D array=w3937, element=w3936) -> (index of element=w3935:i32)  [unwired: 1 out]
            n1562 = Less Than 0?(x=w3935) -> (x < 0?=w3932:bool)
            n1563 = case shown="False" w3932 {
              selector: w3932 -> [_ w3980]
              tunnel: [w3976 w3980] -> w3931
              frame False {
                n1564 = Two Button Dialog(message="There is already on object on the diagram with this name.\nDo you want to add this object anyway?" ("regular expression"), 1:"Cancel" ("regular expression"), 2:"Add object" ("regular expression")) -> (T button?=w3976:bool)
              }
              frame True {
              }
            }
            n1565 = Compound Arithmetic op=AND(TRUE, w3951, w3949, w3931) -> (w3950:bool)
            n1566 = case shown="False" w3950 {
              tunnel: w3975 -> [w3992 w4031]
              tunnel: [w3992 w4030] -> w3974
              tunnel: w3938 -> [w3984 w4029]
              tunnel: w3941 -> [w3985 w4028]
              tunnel: [w3991 w4020] -> w3972
              tunnel: [w3983 w4019] -> w3971
              tunnel: w3940 -> [_ w4018]
              tunnel: w3967 -> [w3981 w4017]
              tunnel: w3965 -> [_ w4014]
              tunnel: w3942 -> [_ w4016]
              tunnel: w3934 -> [w3990 _]
              tunnel: w3933 -> [w3982 _]
              frame False {
                n1567 = call <vilib>:"Check if File or Folder Exists.vi"("path"=w3981) -> ("file or folder exists?"=w3987:bool)  [unwired: 1 in, 9 out]
                n1568 = Equal?(x=diagramType."State" ("diagramType"), y=w3990) -> (x = y?=w3988:bool)
                n1569 = And(x=w3988, y=w3987) -> (x .and. y?=w3986:bool)
                n1570 = case shown="True" w3986 {
                  tunnel: [UMLEditor_statesType."Idle" ("state") UMLEditor_statesType."Repaint" ("state")] -> w3991
                  tunnel: w3985 -> [_ w3999]
                  tunnel: w3984 -> [w3993 w3997]
                  tunnel: [w3993 w4005] -> w3983
                  tunnel: w3982 -> [_ w4003]
                  tunnel: w3981 -> [_ w4000]
                  frame False {
                  }
                  frame True {
                    n1571 = To More Specific Class(target class=refnum<class "StateDiagramGraph.lvclass"> refnum ("reference out"), reference=w3999, error in=w3997) -> (specific class reference=w3998:refnum<class "StateDiagramGraph.lvclass">, error out=w3996:errorcluster)
                    n1572 = Unbundle By Name(w4003) -> ("graphics"=w4002:refnum<class "Graphics.lvclass">, "grid"=w4001:refnum<class "Grid.lvclass">)
                    n1573 = call <resource>:"SetPathInfo.vi"("reference"=w3998, "StateDiagramData.VI-Path"=w4000, "error in (no error)"=w3996) -> ("reference out"=w4007:refnum<class "StateDiagramGraph.lvclass">, "error out"=w4006:errorcluster)  [unwired: 1 in, 14 out]
                    n1574 = call-dynamic "HandleRightClickMenuOption.vi"("reference"=w4007, "MenuOption"="Update diagram...", "graphics"=w4002, "grid"=w4001, "error in (no error)"=w4006) -> ("error out"=w4005:errorcluster)  [unwired: 12 in, 2 out]
                  }
                }
              }
              frame True {
                n1575 = call-dynamic "findNode.vi"("reference"=w4028, "error in (no error)"=w4029) -> ("reference out"=w4015:refnum<class "Graph.lvclass">, "node"=w4027:refnum<class "AbstractNode.lvclass">, "found"=w4026:bool, "error out"=w4022:errorcluster)  [unwired: 14 in]
                n1576 = call <resource>:"UMLEditor ToolBarSettings.vi"("NodeName/EdgeName(empty=not in use)"="ClassNode", "graph(only used with className input)"=w4015, "error in (no error)"=w4022) -> ("prototypeNode"=w4021:refnum<class "AbstractNode.lvclass">, "error out"=w4012:errorcluster)  [unwired: 1 in, 14 out]
                n1577 = call-dynamic "clone.vi"("reference"=w4021, "error in (no error)"=w4012) -> ("clonedAbstractNode"=w4009:refnum<class "AbstractNode.lvclass">, "error out"=w4011:errorcluster)  [unwired: 15 in, 1 out]
                n1578 = call <resource>:"FindFreePosition.vi"("reference"=w4015, "NodePointIn"=w4014, "Node"=w4009, "error in (no error)"=w4011) -> ("NodePointOut"=w4013:T12, "error out"=w4010:errorcluster)  [unwired: 14 out]
                n1579 = call-dynamic "add.vi"("reference"=w4015, "node"=w4009, "point"=w4013, "error in (no error)"=w4010) -> ("added"=w4025:bool, "error out"=w4024:errorcluster)  [unwired: 13 in, 1 out]
                n1580 = case shown="True" w4025 {
                  tunnel: w4031 -> [w4041 w4074]
                  tunnel: [w4040 w4072] -> w4030
                  tunnel: w4024 -> [w4036 w4069]
                  tunnel: w4009 -> [w4034 w4057]
                  tunnel: w4013 -> [w4038 w4070]
                  tunnel: [w4037 w4075] -> w4019
                  tunnel: w4026 -> [w4033 _]
                  tunnel: w4027 -> [w4039 _]
                  tunnel: w4018 -> [_ w4067]
                  tunnel: [UMLEditor_statesType."Idle" ("state") w4066] -> w4020
                  tunnel: w4017 -> [_ w4060]
                  tunnel: w4016 -> [_ w4059]
                  frame False {
                    n1581 = call-dynamic "Destroy.vi"("reference"=w4034, "error in (no error)"=w4036) -> ("error out"=w4035:errorcluster)  [unwired: 16 in, 1 out]
                    n1582 = case shown="True" w4033 {
                      tunnel: w4041 -> [w4042 w4055]
                      tunnel: [w4042 w4054] -> w4040
                      tunnel: w4039 -> [_ w4053]
                      tunnel: w4038 -> [_ w4052]
                      tunnel: [w4043 w4051] -> w4037
                      tunnel: w4035 -> [w4043 w4050]
                      frame False {
                      }
                      frame True {
                        # "Node Found"
